vi "configureRange.vi"(8 "error in (no error)":errorcluster, 11 "ElectrometerController in":refnum<class "ElectrometerController.lvclass">) -> (0 "error out":errorcluster, 2 "Input Range":dbl=10.0 format="%#_10g", 3 "ElectrometerController out":refnum<class "ElectrometerController.lvclass">)   [LabVIEW 2016, in "ElectrometerController.lvclass"]
uses:
  ElectrometerController.lvclass
  Electrometer/Electrometer.lvclass
  ElectrometerConfiguration/ElectrometerInternalConfiguration.lvclass
  Electrometer/State/ElectrometerState.lvclass
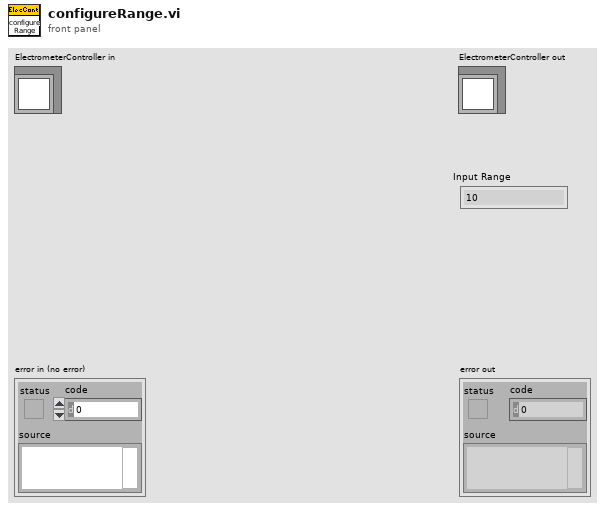
[diagram p1: front panel]
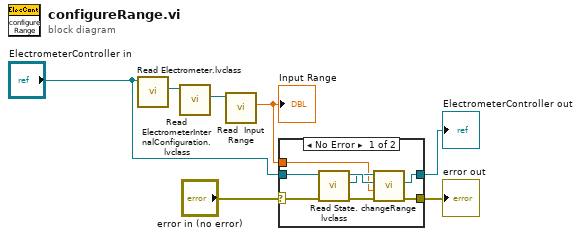
[diagram p0: block diagram]
diagram:
  n1 = call-dynamic "Read Electrometer.lvclass.vi"("ElectrometerController in"="ElectrometerController in") -> ("Electrometer.lvclass"=w3:refnum<class "Electrometer.lvclass">)  [unwired: 8 in, 2 out]
  n2 = call-dynamic "Read ElectrometerInternalConfiguration.lvclass.vi"("Electrometer in"=w3) -> ("ElectrometerInternalConfiguration.lvclass"=w4:refnum<class "ElectrometerInternalConfiguration.lvclass">)  [unwired: 8 in, 2 out]
  n3 = call-dynamic "Read  Input Range .vi"("ElectrometerInternalConfiguration in"=w4) -> ("Input Range"=w1:dbl)  [unwired: 8 in, 2 out]
  "Input Range" <- w1
  n4 = case shown="No Error" "error in (no error)" {
    selector: "error in (no error)" -> [w14 w17]
    tunnel: [w12 w17] -> w6
    tunnel: [w13 w16] -> w5
    tunnel: "ElectrometerController in" -> [w15 w16]
    tunnel: w1 -> [w8 _]
    frame No Error {
      n5 = call-dynamic "Read State.lvclass.vi"("error in (no error)"=w14, "ElectrometerController in"=w15) -> ("error out"=w11:errorcluster, "ElectrometerState"=w9:refnum<class "ElectrometerState.lvclass">, "ElectrometerController out"=w10:refnum<class "ElectrometerController.lvclass">)  [unwired: 7 in]
      n6 = call-dynamic "changeRange.vi"("error in (no error)"=w11, "Input Range"=w8, "ElectrometerController in"=w10, "ElectrometerState in"=w9) -> ("error out"=w12:errorcluster, "ElectrometerController out"=w13:refnum<class "ElectrometerController.lvclass">)  [unwired: 5 in, 1 out]
    }
    frame Error {
    }
  }
  "error out" <- w6
  "ElectrometerController out" <- w5
